vi "ExampleClient.vi"() -> ()   [LabVIEW 2017]
uses:
  jsonRPCwebservice/client/config.ctl
  <vilib>/rvi/Analysis/control/PID/Typedef/niFpgaPID_PIGains.ctl
  <vilib>/rvi/Analysis/control/PID/Typedef/niFpgaPID_OutputRange.ctl
  <vilib>/NI/PowerElectronicsControl/ActiveFrontEnd/AFE/PI_Settings.ctl
  <vilib>/NI/PowerElectronicsControl/Buck-Boost/RealTime/TuningParameters.ctl
  <vilib>/NI/PowerElectronicsControl/Buck-Boost/FPGA/contState.ctl
  Support/StreamClientState.ctl
  Controller/Support/StreamHeader.ctl
  Support/msg.ctl
  <userlib>/_SEH/Controls/CEH/CEH Actions.ctl
  <vilib>/NI/JSON Support for LabVIEW/JSON Data Classes/JSON String/JSON String.lvclass
  C:/Program Files (x86)/National Instruments/LabVIEW 2017/vi.lib/NI/JSON Support for LabVIEW/JSON Data Classes/JSON Datatype/JSON Null.lvclass
  <vilib>/NI/JSON Support for LabVIEW/JSON Data Classes/JSON Object/JSON Object.lvclass
  <vilib>/NI/JSON Support for LabVIEW/JSON Data Classes/JSON Numeric/JSON Numeric.lvclass
  Support/client_globals.vi
  jsonRPCwebservice/client/Request_int_JSON.vi
  <vilib>/NI/JSON Support for LabVIEW/JSON Data Classes/JSON Helper/To More Specific Type (Object).vi
  <vilib>/NI/JSON Support for LabVIEW/JSON Data Classes/JSON String/New JSON String.vi
  <vilib>/NI/JSON Support for LabVIEW/JSON Data Classes/JSON Helper/Parsing/Parse Value.vi
  <vilib>/NI/JSON Support for LabVIEW/JSON Data Classes/JSON Object/Get Value (Array).vi
  <vilib>/NI/JSON Support for LabVIEW/JSON Data Classes/JSON Array/Index Array XNode/index helper.vi
  <vilib>/NI/JSON Support for LabVIEW/JSON Data Classes/JSON Array/Index Array.vi
  <vilib>/NI/JSON Support for LabVIEW/JSON Data Classes/JSON Array/Index Array (JSON).vi
  <vilib>/NI/JSON Support for LabVIEW/JSON Data Classes/JSON Helper/To More Specific Type (Array).vi
  <vilib>/NI/JSON Support for LabVIEW/JSON Data Classes/JSON Array/Get Array Values as Strings.vi
  <vilib>/WebDAVClient/Simple Get File.vi
  <vilib>/NI/JSON Support for LabVIEW/JSON Data Classes/JSON Object/New JSON Object (Multi).vi
  <vilib>/NI/JSON Support for LabVIEW/JSON Data Classes/JSON Numeric/New JSON Numeric.vi
  <vilib>/NI/JSON Support for LabVIEW/JSON Data Classes/JSON Object/Get Value by Array (Object).vi
  <vilib>/NI/JSON Support for LabVIEW/JSON Data Classes/JSON Object/Get Value (Object).vi
  <vilib>/NI/JSON Support for LabVIEW/JSON Data Classes/JSON Datatype/JSON Null.lvclass
  <vilib>/NI/JSON Support for LabVIEW/JSON Data Classes/JSON Array/Index Array XNode/Index JSON Array.xnode
  <vilib>/NI/JSON Support for LabVIEW/JSON Data Classes/JSON Array/JSON Array.lvclass
  jsonRPCwebservice/client/JSON_RPC_client.lvlib
  <vilib>/WebDAVClient/NI_WebDAV.lvlib
  <vilib>/NI/JSON Support for LabVIEW/JSON Data Classes/JSON Helper/JSON Helper.lvclass
  <vilib>/NI/PowerElectronicsControl/ActiveFrontEnd/AFE/ActiveFrontEnd.lvlib
  <vilib>/NI/PowerElectronicsControl/Buck-Boost/FPGA/BuckBoost.lvlib
  <vilib>/NI/PowerElectronicsControl/Buck-Boost/RealTime/BuckBoostInterface.lvlib
panel:
  out "Load Current":dbl format="%_6g"
  out "BuckBoostEnabled":bool
  out "AFE_Enabled":bool
  out "Connected":bool
  out "Fault Registers":u64 format="%016x"
  out "VLoad":dbl format="%_6g"
  out "VDCLink":dbl format="%_6g"
  out "Detected Frequency":dbl format="%1_6g"
  out "locked":bool
  out "UnrecoverableSafeState":bool
  out "SafeState":bool
  out "Powered":bool
  out "EnableBuckBoost":bool
  out "EnableAFE":bool
  out "Precharge":bool
  out "Ready":bool
  out "Synchronize":bool
  out "TuneBuckBoost":bool
  out "TuneAFE":bool
  out "TunePLL":bool
  out "Idle":bool
  out "Initialize":bool
  in  "Connection":T1={"ip"="0.0.0.0", "port"=8001, "username"="admin", "password"=""}
  in  "Trace":string
  in  "Tab Control":T2(tab)
  in  "ClearSafeState":bool
  in  "ToEcho":string
  in  "CheckConnection":bool
  in  "GoToSafeState":bool
  in  "GetResourceUsage":bool
  in  "echo":bool
  out "logging":bool
  out "Waveforms":sgl[][](graph)
  in  "Stream":bool
  in  "StreamAndLog":bool
  in  "StopStreaming":bool
  in  "ForceTigger":bool
  in  "RefreshLogFiles":bool
  in  "Logs":i32(listbox)
  in  "Download":bool
  in  "BuckBoostSetpoint":dbl caption="Setpoint" format="%_6g"
  in  "TurnOffSystem":bool
  in  "SetBuckBoostSetpoint":bool
  in  "TurnOnSystem":bool
  in  "PrechargeSystem":bool
  in  "PLL Range":T3={"output high (Inf)"=inf, "output low (-Inf)"=-inf}
  in  "PLL Gains":T4 {"proportional gain" step=0.125}
  in  "SetPLL_Tune":bool
  in  "GoToTunePLL":bool
  in  "disableAFE":bool
  in  "enableAFE":bool
  in  "SetAFE_tune":bool
  in  "GoToTuneAFE":bool
  in  "IQ_to_VQ":T5={"gains"={"proportional gain"=0.0, "integral gain"=0.0}, "output range"={"output high (Inf)"=inf, "output low (-Inf)"=-inf}, "PI_state"=enum."idle", "reset"=FALSE, "manual"=0.0} {"gains"."proportional gain" step=0.125}
  in  "ID_to_VD":T5={"gains"={"proportional gain"=0.0, "integral gain"=0.0}, "output range"={"output high (Inf)"=inf, "output low (-Inf)"=-inf}, "PI_state"=enum."idle", "reset"=FALSE, "manual"=0.0} {"gains"."proportional gain" step=0.125}
  in  "VDCLinkToPower":T5={"gains"={"proportional gain"=0.0, "integral gain"=0.0}, "output range"={"output high (Inf)"=inf, "output low (-Inf)"=-inf}, "PI_state"=enum."idle", "reset"=FALSE, "manual"=0.0} {"gains"."proportional gain" step=0.125}
  in  "disableBuckBoost":bool
  in  "SetBuckBoostTune":bool
  in  "GoToTuneBuckBoost":bool
  in  "CompleteTuning":bool
  in  "BuckBoostTune":T6 caption="Buck-Boost Tune" {"gains"."proportional gain" step=0.125}
  in  "enableBuckBoost":bool
  in  "Exit":bool
  # "Tuning"
  # "rad/sec"
  # "V"
  # "V"
  # "Amps"
  # "Amps"
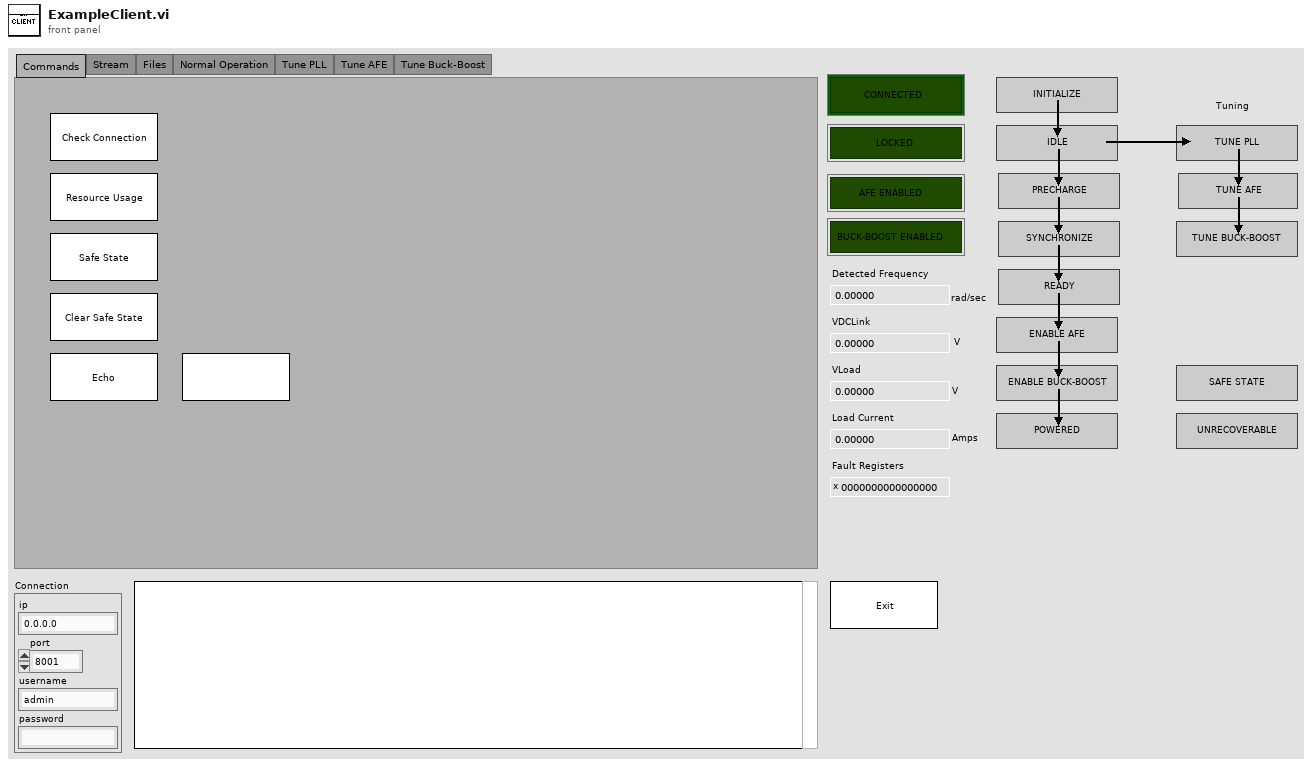
[diagram p1: front panel]
types:
  T1 = typedef "JSON_RPC_client.lvlib/config.ctl" = cluster{"ip":string, "port":i32, "username":string, "password":string}
  T2 = enum32{"Commands", "Stream", "Files", "Normal Operation", "Tune PLL", "Tune AFE", "Tune Buck-Boost"}
  T3 = typedef "niFpgaPID_OutputRange.ctl" = cluster{"output high (Inf)":sgl, "output low (-Inf)":sgl}
  T4 = typedef "niFpgaPID_PIGains.ctl" = cluster{"proportional gain":sgl, "integral gain":sgl}
  T5 = typedef "ActiveFrontEnd.lvlib/PI_Settings.ctl" = cluster{"gains":T4, "output range":T3, "PI_state":enum8{"idle", "normal", "manual", "perturbance"}, "reset":bool, "manual":sgl}
  T6 = typedef "BuckBoostInterface.lvlib/TuningParameters.ctl" = cluster{"gains":T4, "manualInput":sgl, "rampRate":sgl, "pertAmp":sgl, "pertFreq":sgl, "controlFreq":sgl, "state":T7}
  T7 = typedef "BuckBoost.lvlib/contState.ctl" = enum16{"disabled", "manual", "normal", "perturb"}
  T8 = typedef "msg.ctl" = cluster{"cmd":string, "parameters":variant}
  T9 = typedef "StreamHeader.ctl" = cluster{"Channels":string[], "SampleRate":i32}
  T10 = typedef "StreamClientState.ctl" = enum16{"Initialize", "Idle", "ConnectAndOpen", "Connecting", "ReadHeader", "Streaming", "Disconnecting"}
  T11 = enum8{"Enabled", "Disabled", "Disabled and Grayed Out"}
  T12 = typedef "JSON_RPC_client.lvlib/reference.ctl" = cluster{"client handle":T13, "url":string}
  T13 = typedef "LabVIEWHTTPClient.lvlib/ClientHandle.ctl" = refnum<k1>
  T14 = typedef "StateMsg.ctl" = cluster{"State":string, "locked":bool, "DetectedFrequency":dbl, "VDCLink":dbl, "VLoad":dbl, "FaultRegisters":u64, "afeEnabled":bool, "buckboostEnabled":bool, "LoadCurrent":dbl}
  T15 = typedef "SEH Notification Info.ctl" = cluster{"Priority":i32, "Occurrences":i32, "First Occurrence":timestamp}
  T16 = typedef "CEH Actions.ctl" = enum16{"Log", "Display Error Message", "Safe State", "Shutdown"}
  T17 = enum16{"open", "open or create", "create or replace", "create", "open (read-only)"}
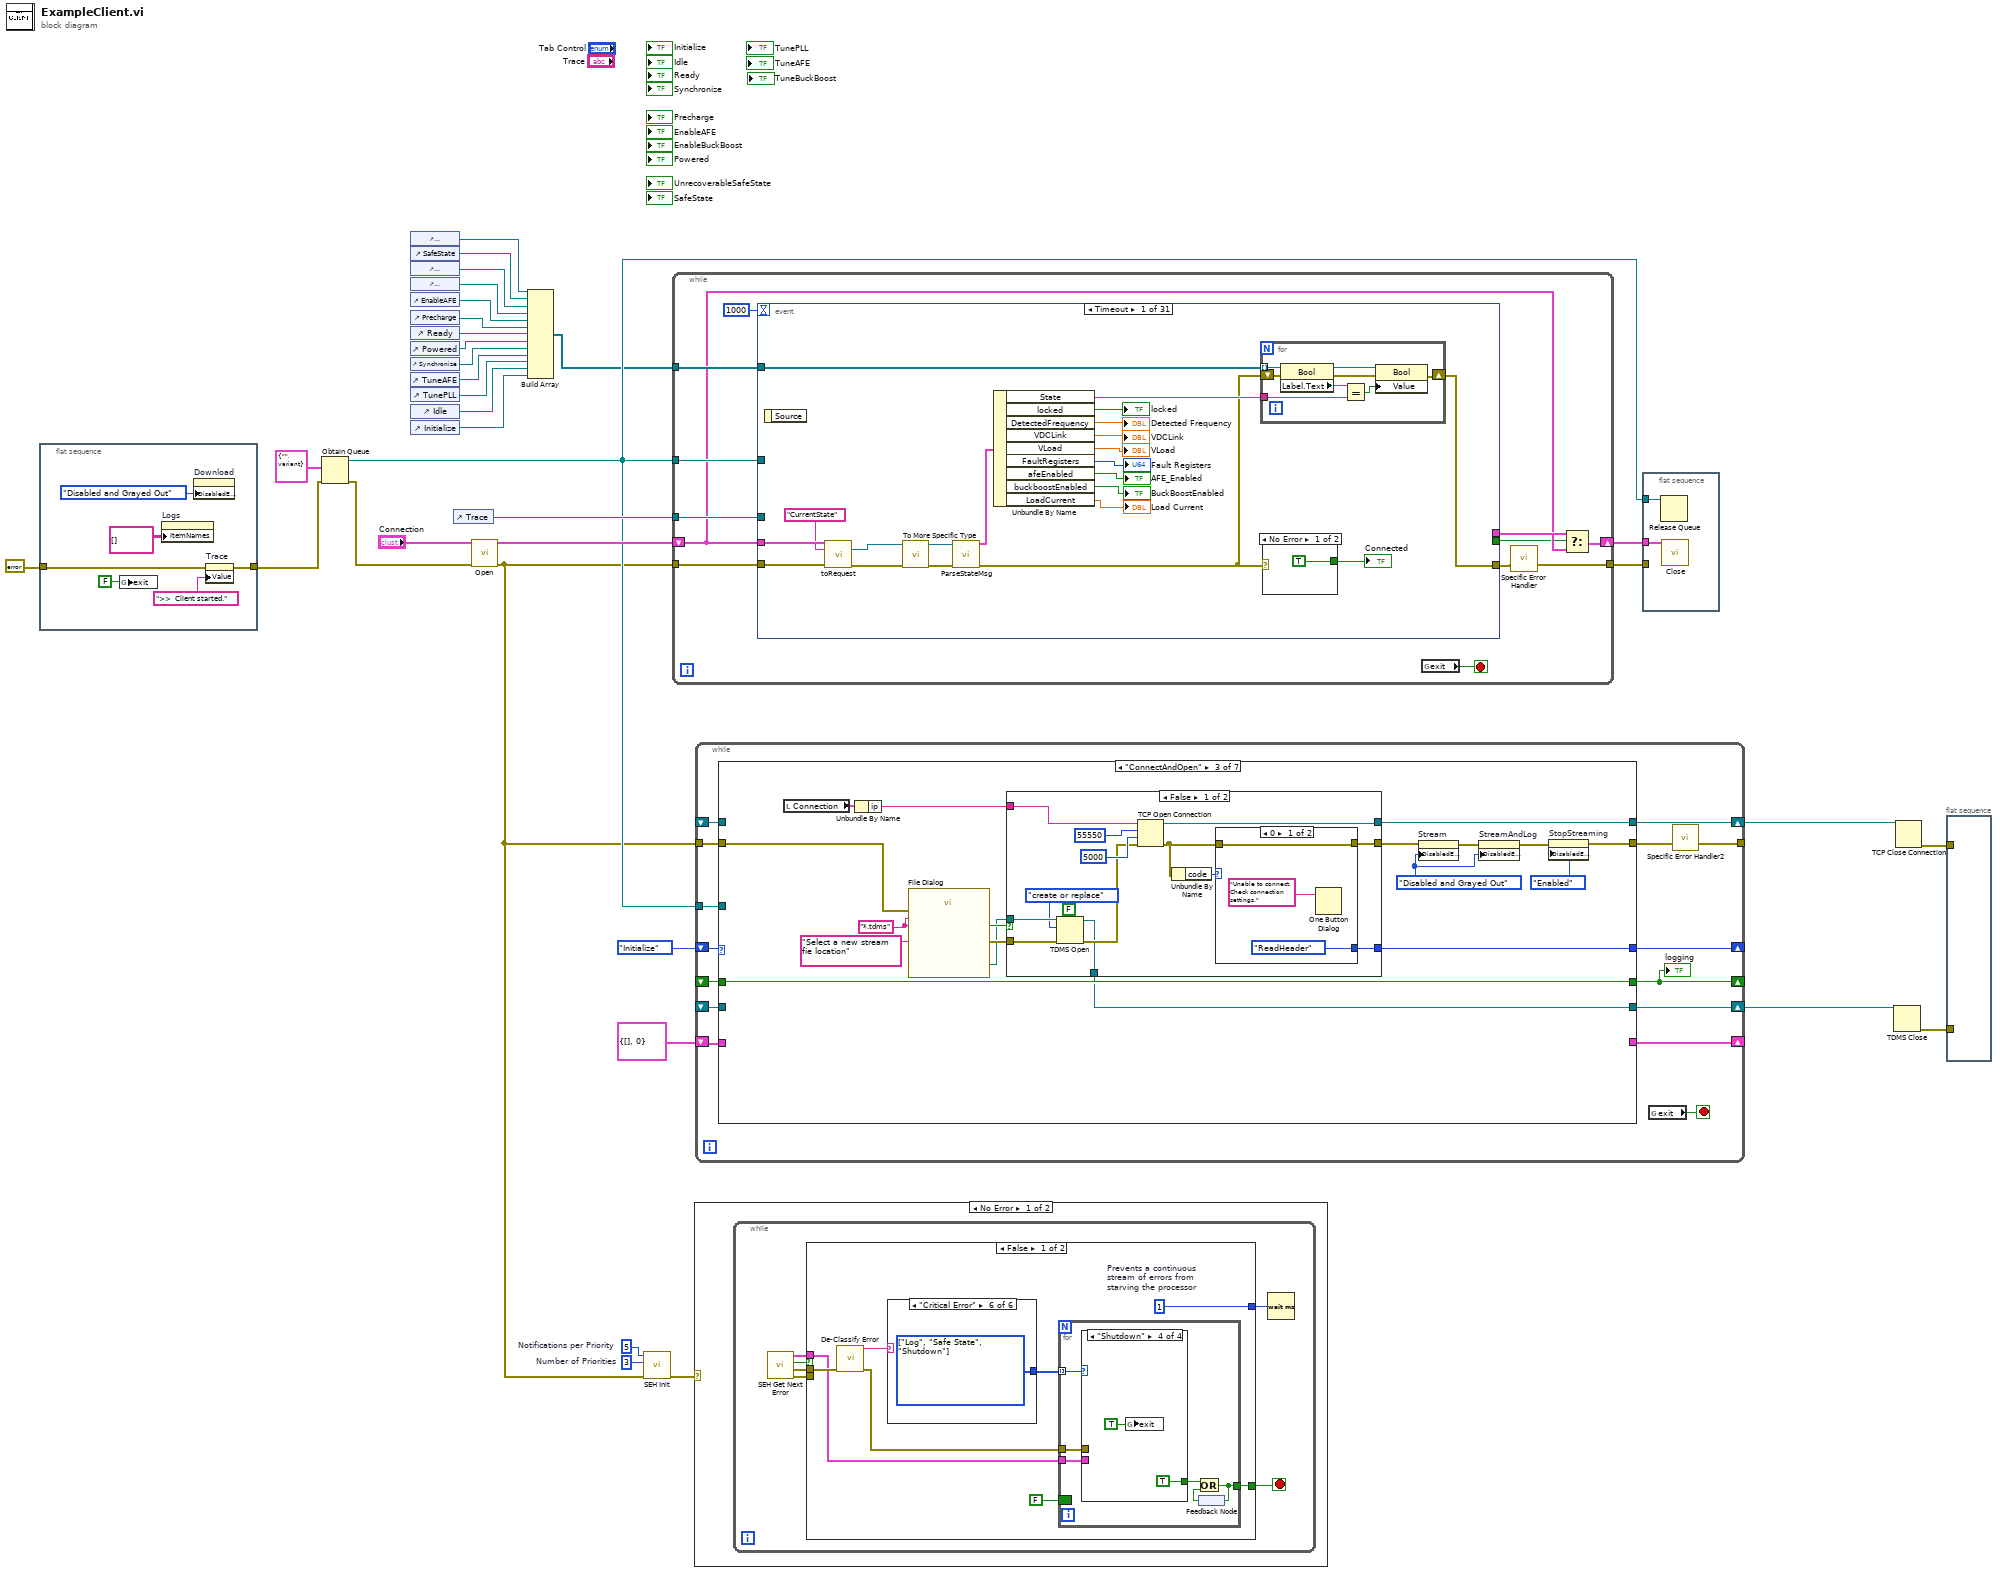
[diagram p0: block diagram]
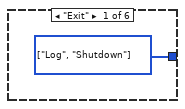
[diagram p2: hidden frame]
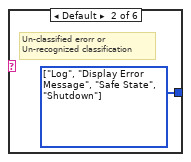
[diagram p3: hidden frame]
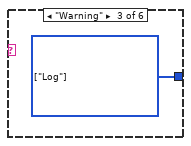
[diagram p4: hidden frame]
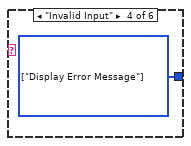
[diagram p5: hidden frame]
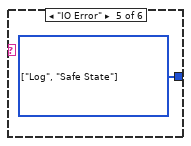
[diagram p6: hidden frame]
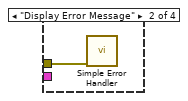
[diagram p8: hidden frame]
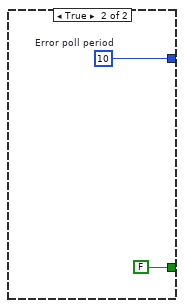
[diagram p10: hidden frame]
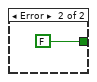
[diagram p12: hidden frame]
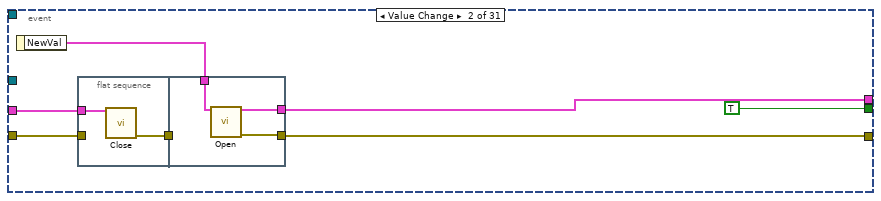
[diagram p13: hidden frame]
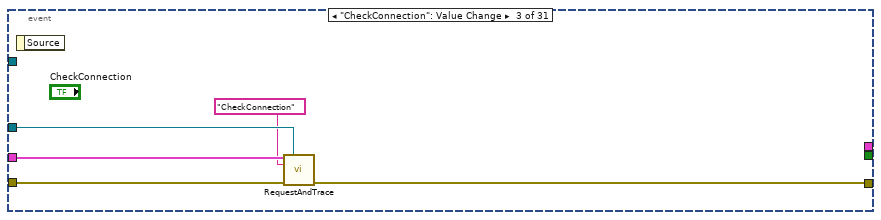
[diagram p14: hidden frame]
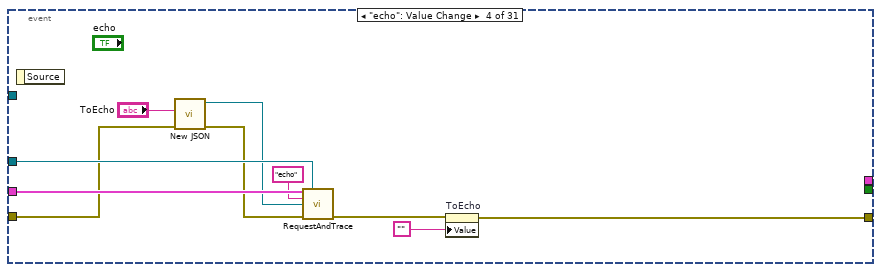
[diagram p15: hidden frame]
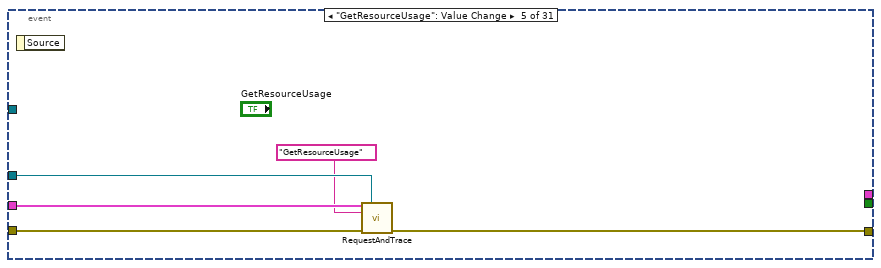
[diagram p16: hidden frame]
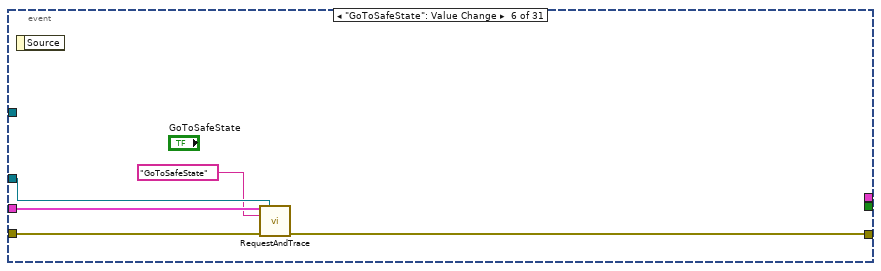
[diagram p17: hidden frame]
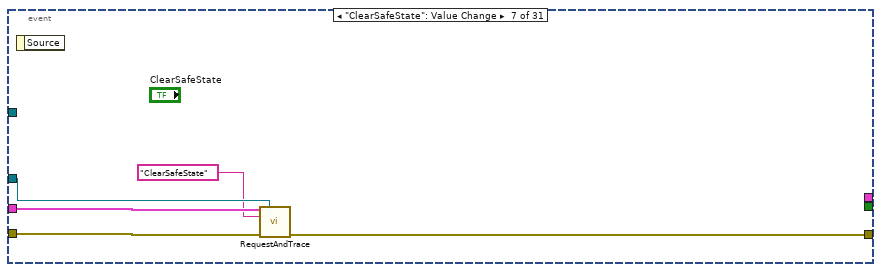
[diagram p18: hidden frame]
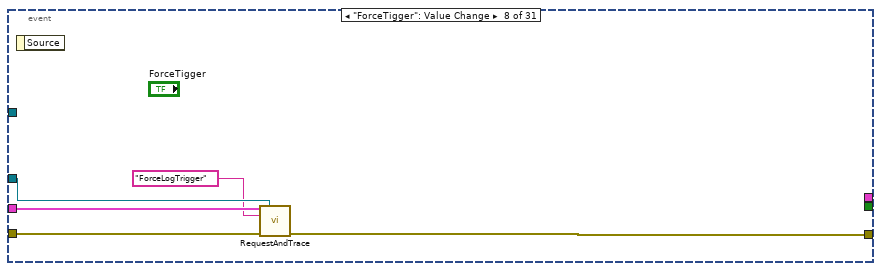
[diagram p19: hidden frame]
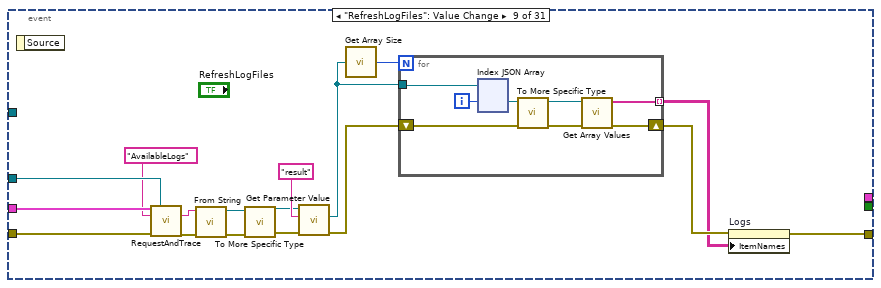
[diagram p20: hidden frame]
diagram:
  w23 = 3  # Number of Priorities
  w22 = 5  # Notifications per Priority
  n1 = flat-sequence {
    tunnel: errorcluster {"status"=FALSE, "code"=0, "source"=""} ("error in (no error)") -> [w38]
    tunnel: [w37] -> w27
    frame #0 {
      n2 = global write "client_globals.vi" "exit"(FALSE ("exit")) -> ()
      n3 = property on="Logs" class="MCListbox (strict)"("ItemNames"=string[][] [] ("Item Names")) -> ()  [unwired: 2 in, 2 out]
      n4 = property on="Download" class="Bool"("DisabledEnum"=T11."Disabled and Grayed Out" ("Disabled")) -> ()  [unwired: 2 in, 2 out]
      n5 = property on="Trace" class="Str"(error in=w38, "Value"=">>  Client started." ("Trace")) -> (error out=w37:errorcluster)  [unwired: 1 in, 1 out]
    }
  }
  n6 = Obtain Queue(element data type=T8 {"cmd"="", "parameters"=variant} ("msg"), error in (no error)=w27) -> (queue out=w25:refnum<queue>, error out=w26:errorcluster)  [unwired: 3 in, 1 out]
  n7 = control-ref of="UnrecoverableSafeState"() -> (w15:refnum<vi>)
  n8 = control-ref of="SafeState"() -> (w14:refnum<vi>)
  n9 = control-ref of="TuneBuckBoost"() -> (w13:refnum<vi>)
  n10 = control-ref of="EnableBuckBoost"() -> (w12:refnum<vi>)
  n11 = control-ref of="EnableAFE"() -> (w11:refnum<vi>)
  n12 = control-ref of="Precharge"() -> (w10:refnum<vi>)
  n13 = control-ref of="Ready"() -> (w9:refnum<vi>)
  n14 = control-ref of="Powered"() -> (w8:refnum<vi>)
  n15 = control-ref of="Synchronize"() -> (w7:refnum<vi>)
  n16 = control-ref of="TuneAFE"() -> (w6:refnum<vi>)
  n17 = control-ref of="TunePLL"() -> (w5:refnum<vi>)
  n18 = control-ref of="Idle"() -> (w4:refnum<vi>)
  n19 = control-ref of="Initialize"() -> (w3:refnum<vi>)
  n20 = control-ref of="Trace"() -> (w29:refnum<vi>)
  n21 = call "Open.vi"("config"="Connection", "error in (no error)"=w26) -> ("reference"=w32:T12, "error out"=w20:errorcluster)  [unwired: 12 in]
  n22 = Build Array(w15, w14, w13, w12, w11, w10, w9, w8, w7, w6, w5, w4, w3) -> (w2:refnum<vi>[])
  n23 = call <userlib>:"SEH Init.vi"("error in (no error)"=w20, "Number of Priorities"=w23, "Notifications per Priority"=w22) -> ("error out"=w21:errorcluster)  [unwired: 8 in]
  n24 = while {
    tunnel: w29 -> [w47]
    tunnel: w25 -> [w46]
    tunnel: w20 -> [w52]
    tunnel: [w48] -> w30
    tunnel: w2 -> [w45]
    shift-right: [w44] -> w1
    shift-left: w32 -> [w42]
    stop <- w50 stop-if-true
    n25 = event shown="[0] Timeout" {
      selector: _ -> [_ _ _ _ _ _ _ _ _ _ _ _ _ _ _ _ _ _ _ _ _ _ _ _ _ _ _ _ _ _ _]
      dyn-events: _ -> [_ _ _ _ _ _ _ _ _ _ _ _ _ _ _ _ _ _ _ _ _ _ _ _ _ _ _ _ _ _ _]
      timeout: 1000 -> [_ _ _ _ _ _ _ _ _ _ _ _ _ _ _ _ _ _ _ _ _ _ _ _ _ _ _ _ _ _ _]
      tunnel: w42 -> [w72 w90 w98 w110 w115 w120 w125 w130 w147 _ _ _ _ _ w216 w221 w226 w231 w236 w241 w257 w265 w269 w288 w293 w298 w303 w308 w316 w322 _]
      tunnel: w52 -> [w73 w89 w100 w103 w114 w119 w124 w129 w146 w163 w183 w198 w204 w211 w217 w222 w227 w232 w237 w242 w246 w261 w270 w284 w290 w295 w300 w305 w313 w319 _]
      tunnel: [w67 w85 w99 w107 w112 w117 w122 w127 w144 w164 w176 w197 w201 w207 w215 w220 w225 w230 w235 w240 w256 w264 w268 w287 w292 w297 w302 w307 w315 w321 errorcluster {"status"=TRUE, "code"=-1, "source"="User selected exit."} ("error out")] -> w49
      tunnel: w47 -> [_ _ w97 w109 w113 w118 w123 w128 w145 _ _ _ w200 w209 w214 w219 w224 w229 w234 w239 w255 w263 w267 w286 w291 w296 w301 w306 w314 w320 _]
      tunnel: w46 -> [_ _ _ _ _ _ _ _ _ _ _ w199 w205 w212 _ _ _ _ _ _ _ _ _ _ _ _ _ _ _ _ _]
      tunnel: w45 -> [w68 _ _ _ _ _ _ _ _ _ _ _ _ _ _ _ _ _ _ _ _ _ _ _ _ _ _ _ _ _ _]
      tunnel: [_ w86 _ _ _ _ _ _ _ _ _ _ _ _ _ _ _ _ _ _ _ _ _ _ _ _ _ _ _ _ _] -> w43
      tunnel: [_ TRUE _ _ _ _ _ _ _ _ _ _ _ _ _ _ _ _ _ _ _ _ _ _ _ _ _ _ _ _ _] -> w41
      event Timeout {
        n26 = event-data() -> ()  [unwired: 1 in, 1 out]
        n27 = call-poly "toRequest.vi"("reference in"=w72, "method"="CurrentState" ("resulting string"), "error in (no error)"=w73) -> ("response"=w70:refnum<class "JSON Null.lvclass">, "error out"=w69:errorcluster)  [unwired: 10 in, 1 out]
        n28 = call-poly <vilib>:"To More Specific Type.vi"("error in (no error)"=w69, "JSON Datatype in"=w70) -> ("error out"=w65:errorcluster, "JSON Datatype out"=w64:refnum<class "JSON Object.lvclass">)  [unwired: 8 in]
        n29 = call "ParseStateMsg.vi"("StateMsg"=w64, "error in"=w65) -> ("StateMsg"=w63:T14, "error out"=w61:errorcluster)  [unwired: 12 in]
        n30 = Unbundle By Name(w63) -> ("State"=w62:string, "locked"=→"locked":bool, "DetectedFrequency"=→"Detected Frequency":dbl, "VDCLink"=→"VDCLink":dbl, "VLoad"=→"VLoad":dbl, "FaultRegisters"=→"Fault Registers":u64, "afeEnabled"=→"AFE_Enabled":bool, "buckboostEnabled"=→"BuckBoostEnabled":bool, "LoadCurrent"=→"Load Current":dbl)
        n31 = for {
          tunnel: w62 -> [w81]
          tunnel: w68 -> [w83] mode=indexing
          shift-right: [w77] -> w67
          shift-left: w61 -> [w78]
          n32 = property class="Bool"(reference=w83, error in=w78) -> (reference out=w80:refnum<vi>, error out=w76:errorcluster, "Label.Text"=w82:string)
          n33 = Equal?(x=w82, y=w81) -> (x = y?=w79:bool)
          n34 = property class="Bool"(reference=w80, error in=w76, "Value"=w79) -> (error out=w77:errorcluster)  [unwired: 1 out]
        }
        n35 = case shown="No Error" w61 {
          tunnel: [TRUE FALSE] -> w66
          frame No Error {
          }
          frame Error {
          }
        }
        "Connected" <- w66
      }
      event Value Change {
        n36 = event-data() -> ("NewVal"=w87:T1)  [unwired: 1 in]
        n37 = flat-sequence {
          tunnel: w90 -> [w92]
          tunnel: w89 -> [_]
          tunnel: [w91] -> w88
          tunnel: w88 -> [_]
          tunnel: w87 -> [w95]
          tunnel: [w94] -> w85
          tunnel: [w93] -> w86
          frame #0 {
            n38 = call "Close.vi"("reference in"=w92) -> ("error out"=w91:errorcluster)  [unwired: 14 in]
          }
          frame #1 {
            n39 = call "Open.vi"("config"=w95) -> ("reference"=w93:T12, "error out"=w94:errorcluster)  [unwired: 13 in]
          }
        }
      }
      event "CheckConnection": Value Change {
        n40 = event-data() -> ()  [unwired: 1 in, 1 out]
        n41 = call "RequestAndTrace.vi"("JSONRef in"=w98, "TraceRef"=w97, "method"="CheckConnection" ("resulting string"), "error in (no error)"=w100) -> ("error out"=w99:errorcluster)  [unwired: 9 in, 2 out]
      }
      event "echo": Value Change {
        n42 = event-data() -> ()  [unwired: 1 in, 1 out]
        n43 = call-poly <vilib>:"New JSON.vi"("error in (no error)"=w103, "value"="ToEcho") -> ("error out"=w102:errorcluster, "JSON String out"=w101:refnum<class "JSON String.lvclass">)  [unwired: 8 in]
        n44 = call "RequestAndTrace.vi"("JSONRef in"=w110, "TraceRef"=w109, "method"="echo" ("resulting string"), "params"=w101, "error in (no error)"=w102) -> ("error out"=w108:errorcluster)  [unwired: 8 in, 2 out]
        n45 = property on="ToEcho" class="Str"(error in=w108, "Value"="") -> (error out=w107:errorcluster)  [unwired: 1 in, 1 out]
      }
      event "GetResourceUsage": Value Change {
        n46 = event-data() -> ()  [unwired: 1 in, 1 out]
        n47 = call "RequestAndTrace.vi"("JSONRef in"=w115, "TraceRef"=w113, "method"="GetResourceUsage" ("resulting string"), "error in (no error)"=w114) -> ("error out"=w112:errorcluster)  [unwired: 9 in, 2 out]
      }
      event "GoToSafeState": Value Change {
        n48 = event-data() -> ()  [unwired: 1 in, 1 out]
        n49 = call "RequestAndTrace.vi"("JSONRef in"=w120, "TraceRef"=w118, "method"="GoToSafeState" ("resulting string"), "error in (no error)"=w119) -> ("error out"=w117:errorcluster)  [unwired: 9 in, 2 out]
      }
      event "ClearSafeState": Value Change {
        n50 = event-data() -> ()  [unwired: 1 in, 1 out]
        n51 = call "RequestAndTrace.vi"("JSONRef in"=w125, "TraceRef"=w123, "method"="ClearSafeState" ("resulting string"), "error in (no error)"=w124) -> ("error out"=w122:errorcluster)  [unwired: 9 in, 2 out]
      }
      event "ForceTigger": Value Change {
        n52 = event-data() -> ()  [unwired: 1 in, 1 out]
        n53 = call "RequestAndTrace.vi"("JSONRef in"=w130, "TraceRef"=w128, "method"="ForceLogTrigger" ("resulting string"), "error in (no error)"=w129) -> ("error out"=w127:errorcluster)  [unwired: 9 in, 2 out]
      }
      event "RefreshLogFiles": Value Change {
        n54 = event-data() -> ()  [unwired: 1 in, 1 out]
        n55 = call "RequestAndTrace.vi"("JSONRef in"=w147, "TraceRef"=w145, "method"="AvailableLogs" ("resulting string"), "error in (no error)"=w146) -> ("reponse"=w141:string, "error out"=w142:errorcluster)  [unwired: 9 in, 1 out]
        n56 = call <vilib>:"From String.vi"("error in (no error)"=w142, "JSON String"=w141) -> ("error out"=w134:errorcluster, "JSON out"=w133:refnum<class "JSON Null.lvclass">)  [unwired: 8 in]
        n57 = call-poly <vilib>:"To More Specific Type.vi"("error in (no error)"=w134, "JSON Datatype in"=w133) -> ("error out"=w131:errorcluster, "JSON Datatype out"=w132:refnum<class "JSON Object.lvclass">)  [unwired: 8 in]
        n58 = call-poly <vilib>:"Get Parameter Value.vi"("error in (no error)"=w131, "key"="result" ("Parameter Name"), "JSON Object in"=w132) -> ("error out"=w139:errorcluster, "value"=w136:refnum<class "JSON Array.lvclass">)  [unwired: 7 in]
        n59 = call <vilib>:"Get Array Size.vi"("JSON Array in"=w136) -> ("size(s)"=w137:i32)
        n60 = for {
          N: w137 -> [_]
          tunnel: w136 -> [w155]
          shift-right: [w149] -> w138
          shift-left: w139 -> [w152]
          tunnel: [w148] -> w135 mode=indexing
          i -> [w154]
          n61 = xnode "Index JSON Array"("index"=w154, "JSON Array In"=w155) -> ("element"=w153:refnum<class "JSON Null.lvclass">)  [unwired: 1 in, 1 out]
          n62 = call-poly <vilib>:"To More Specific Type.vi"("error in (no error)"=w152, "JSON Datatype in"=w153) -> ("error out"=w150:errorcluster, "JSON Datatype out"=w151:refnum<class "JSON Array.lvclass">)  [unwired: 8 in]
          n63 = call-poly <vilib>:"Get Array Values.vi"("error in (no error)"=w150, "JSON Array in"=w151) -> ("error out"=w149:errorcluster, "values"=w148:string[])  [unwired: 8 in]
        }
        n64 = property on="Logs" class="MCListbox (strict)"(error in=w138, "ItemNames"=w135) -> (error out=w144:errorcluster)  [unwired: 1 in, 1 out]
      }
      event "Logs": Value Change {
        n65 = event-data() -> ()  [unwired: 1 in, 1 out]
        n66 = case shown="-1" "Logs" {
          tunnel: w163 -> [w167 w168]
          tunnel: [w167 w168] -> w162
          tunnel: [T11."Enabled" ("Disabled") T11."Disabled and Grayed Out" ("Disabled")] -> w161
          frame Default {
          }
          frame -1 {
          }
        }
        n67 = property on="Download" class="Bool"(error in=w162, "DisabledEnum"=w161) -> (error out=w164:errorcluster)  [unwired: 1 in, 1 out]
      }
      event "Download": Value Change {
        # "http[s]://hostname[:port][/files][/directory/subdirectory]/filename"
        n68 = event-data() -> ()  [unwired: 1 in, 1 out]
        n69 = property on="Logs" class="MCListbox (strict)"() -> ("ItemNames"=w181:string[][])  [unwired: 2 in, 2 out]
        n70 = local read "Connection"() -> (w170:T1)
        n71 = property on="Logs" class="MCListbox (strict)"(error in=w183) -> (error out=w175:errorcluster, "FocusRow"=w182:i32)  [unwired: 1 in, 1 out]
        n72 = Index Array(array=w181, index (row)=w182, index (col)=0 ("index")) -> (element=w173:string)
        n73 = Unbundle By Name(w170) -> ("ip"=w179:string, "username"=w178:string, "password"=w177:string)
        n74 = call "File Dialog2"("error in"=w175) -> ("selected path"=w174:path, "cancelled"=w171:bool, "error out"=w172:errorcluster)  [unwired: 11 in, 1 out]
        n75 = case shown="False" w171 {
          tunnel: w179 -> [w193 _]
          tunnel: w178 -> [w190 _]
          tunnel: w177 -> [w189 _]
          tunnel: [w188 w195] -> w176
          tunnel: w174 -> [w187 _]
          tunnel: w173 -> [w186 _]
          tunnel: w172 -> [w184 w195]
          frame False {
            n76 = Build Path(base path=w187, name or relative path=w186) -> (appended path=w185:path)
            n77 = Concatenate Strings("http://" ("string"), w193, "/files/home/lvuser/logs/" ("string"), w186) -> (w191:string)
            n78 = call-poly <vilib>:"Simple Get.vi"("remote file uri"=w191, "username"=w190, "password"=w189, "local file path"=w185, "error in (no error)"=w184) -> ("error out"=w188:errorcluster)  [unwired: 9 in, 1 out]
          }
          frame True {
          }
        }
      }
      event "Stream": Value Change {
        n79 = event-data() -> ()  [unwired: 1 in, 1 out]
        n80 = Enqueue Element(queue=w199, element=T8 {"cmd"="StartStream", "parameters"=variant}, error in (no error)=w198) -> (error out=w197:errorcluster)  [unwired: 1 in, 2 out]
      }
      event "StreamAndLog": Value Change {
        n81 = event-data() -> ()  [unwired: 1 in, 1 out]
        n82 = Enqueue Element(queue=w205, element=T8 {"cmd"="StartStreamAndLog", "parameters"=variant}, error in (no error)=w204) -> (error out=w202:errorcluster)  [unwired: 1 in, 2 out]
        n83 = call "ToTrace.vi"("ToTrace"="Stream and log started.", "TraceRef"=w200, "error in (no error)"=w202) -> ("error out"=w201:errorcluster)  [unwired: 12 in]
      }
      event "StopStreaming": Value Change {
        n84 = event-data() -> ()  [unwired: 1 in, 1 out]
        n85 = Enqueue Element(queue=w212, element=T8 {"cmd"="StopStream", "parameters"=variant}, error in (no error)=w211) -> (error out=w210:errorcluster)  [unwired: 1 in, 2 out]
        n86 = call "ToTrace.vi"("ToTrace"="Streaming stopped.", "TraceRef"=w209, "error in (no error)"=w210) -> ("error out"=w207:errorcluster)  [unwired: 12 in]
      }
      event "GoToTuneAFE": Value Change {
        n87 = event-data() -> ()  [unwired: 1 in, 1 out]
        n88 = call "RequestAndTrace.vi"("JSONRef in"=w216, "TraceRef"=w214, "method"="GoToTuneAFE" ("resulting string"), "error in (no error)"=w217) -> ("error out"=w215:errorcluster)  [unwired: 9 in, 2 out]
      }
      event "GoToTunePLL": Value Change {
        n89 = event-data() -> ()  [unwired: 1 in, 1 out]
        n90 = call "RequestAndTrace.vi"("JSONRef in"=w221, "TraceRef"=w219, "method"="GoToTunePLL" ("resulting string"), "error in (no error)"=w222) -> ("error out"=w220:errorcluster)  [unwired: 9 in, 2 out]
      }
      event "GoToTuneBuckBoost": Value Change {
        n91 = event-data() -> ()  [unwired: 1 in, 1 out]
        n92 = call "RequestAndTrace.vi"("JSONRef in"=w226, "TraceRef"=w224, "method"="GoToTuneBuckBoost" ("resulting string"), "error in (no error)"=w227) -> ("error out"=w225:errorcluster)  [unwired: 9 in, 2 out]
      }
      event "TurnOnSystem": Value Change {
        n93 = event-data() -> ()  [unwired: 1 in, 1 out]
        n94 = call "RequestAndTrace.vi"("JSONRef in"=w231, "TraceRef"=w229, "method"="TurnOnSystem" ("resulting string"), "error in (no error)"=w232) -> ("error out"=w230:errorcluster)  [unwired: 9 in, 2 out]
      }
      event "TurnOffSystem": Value Change {
        n95 = event-data() -> ()  [unwired: 1 in, 1 out]
        n96 = call "RequestAndTrace.vi"("JSONRef in"=w236, "TraceRef"=w234, "method"="TurnOffSystem" ("resulting string"), "error in (no error)"=w237) -> ("error out"=w235:errorcluster)  [unwired: 9 in, 2 out]
      }
      event "PrechargeSystem": Value Change {
        n97 = event-data() -> ()  [unwired: 1 in, 1 out]
        n98 = call "RequestAndTrace.vi"("JSONRef in"=w241, "TraceRef"=w239, "method"="PrechargeSystem" ("resulting string"), "error in (no error)"=w242) -> ("error out"=w240:errorcluster)  [unwired: 9 in, 2 out]
      }
      event "SetPLL_Tune": Value Change {
        n99 = event-data() -> ()  [unwired: 1 in, 1 out]
        n100 = call <vilib>:"From Variant.vi"("error in (no error)"=w246, "Variant"="PLL Range") -> ("error out"=w254:errorcluster, "JSON out"=w253:refnum<class "JSON Null.lvclass">)  [unwired: 8 in]
        n101 = call <vilib>:"From Variant.vi"("error in (no error)"=w254, "Variant"="PLL Gains") -> ("error out"=w248:errorcluster, "JSON out"=w252:refnum<class "JSON Null.lvclass">)  [unwired: 8 in]
        n102 = Build Array(w253, w252) -> (w251:refnum<class "JSON Null.lvclass">[])
        n103 = call-poly <vilib>:"New JSON.vi"("keys"=string[] ["PLLrange", "PLLgains"], "error in (no error)"=w248, "values"=w251) -> ("error out"=w245:errorcluster, "JSON Object out"=w244:refnum<class "JSON Object.lvclass">)  [unwired: 7 in]
        n104 = call "RequestAndTrace.vi"("JSONRef in"=w257, "TraceRef"=w255, "method"="SetPLL_Tune" ("resulting string"), "params"=w244, "error in (no error)"=w245) -> ("error out"=w256:errorcluster)  [unwired: 8 in, 2 out]
      }
      event "SetBuckBoostSetpoint": Value Change {
        n105 = event-data() -> ()  [unwired: 1 in, 1 out]
        n106 = call-poly <vilib>:"New JSON.vi"("error in (no error)"=w261, "value"="BuckBoostSetpoint") -> ("error out"=w259:errorcluster, "JSON String out"=w260:refnum<class "JSON Numeric.lvclass">)  [unwired: 8 in]
        n107 = call "RequestAndTrace.vi"("JSONRef in"=w265, "TraceRef"=w263, "method"="SetBuckBoostSetpoint" ("resulting string"), "params"=w260, "error in (no error)"=w259) -> ("error out"=w264:errorcluster)  [unwired: 8 in, 2 out]
      }
      event "CompleteTuning": Value Change {
        n108 = event-data() -> ()  [unwired: 1 in, 1 out]
        n109 = call "RequestAndTrace.vi"("JSONRef in"=w269, "TraceRef"=w267, "method"="CompleteTuning" ("resulting string"), "error in (no error)"=w270) -> ("error out"=w268:errorcluster)  [unwired: 9 in, 2 out]
      }
      event "SetAFE_tune": Value Change {
        n110 = event-data() -> ()  [unwired: 1 in, 1 out]
        n111 = call <vilib>:"From Variant.vi"("error in (no error)"=w284, "Variant"="ID_to_VD") -> ("error out"=w283:errorcluster, "JSON out"=w279:refnum<class "JSON Null.lvclass">)  [unwired: 8 in]
        n112 = call <vilib>:"From Variant.vi"("error in (no error)"=w283, "Variant"="IQ_to_VQ") -> ("error out"=w281:errorcluster, "JSON out"=w278:refnum<class "JSON Null.lvclass">)  [unwired: 8 in]
        n113 = call <vilib>:"From Variant.vi"("error in (no error)"=w281, "Variant"="VDCLinkToPower") -> ("error out"=w274:errorcluster, "JSON out"=w277:refnum<class "JSON Null.lvclass">)  [unwired: 8 in]
        n114 = Build Array(w279, w278, w277) -> (w276:refnum<class "JSON Null.lvclass">[])
        n115 = call-poly <vilib>:"New JSON.vi"("keys"=string[] ["ID_to_VD", "IQ_to_VQ", "VDCLinkToPower"], "error in (no error)"=w274, "values"=w276) -> ("error out"=w273:errorcluster, "JSON Object out"=w272:refnum<class "JSON Object.lvclass">)  [unwired: 7 in]
        n116 = call "RequestAndTrace.vi"("JSONRef in"=w288, "TraceRef"=w286, "method"="SetAFE_tune" ("resulting string"), "params"=w272, "error in (no error)"=w273) -> ("error out"=w287:errorcluster)  [unwired: 8 in, 2 out]
      }
      event "enableAFE": Value Change {
        n117 = event-data() -> ()  [unwired: 1 in, 1 out]
        n118 = call "RequestAndTrace.vi"("JSONRef in"=w293, "TraceRef"=w291, "method"="enableAfe" ("resulting string"), "error in (no error)"=w290) -> ("error out"=w292:errorcluster)  [unwired: 9 in, 2 out]
      }
      event "disableAFE": Value Change {
        n119 = event-data() -> ()  [unwired: 1 in, 1 out]
        n120 = call "RequestAndTrace.vi"("JSONRef in"=w298, "TraceRef"=w296, "method"="disableAfe" ("resulting string"), "error in (no error)"=w295) -> ("error out"=w297:errorcluster)  [unwired: 9 in, 2 out]
      }
      event "enableBuckBoost": Value Change {
        n121 = event-data() -> ()  [unwired: 1 in, 1 out]
        n122 = call "RequestAndTrace.vi"("JSONRef in"=w303, "TraceRef"=w301, "method"="enableBuckBoost" ("resulting string"), "error in (no error)"=w300) -> ("error out"=w302:errorcluster)  [unwired: 9 in, 2 out]
      }
      event "disableBuckBoost": Value Change {
        n123 = event-data() -> ()  [unwired: 1 in, 1 out]
        n124 = call "RequestAndTrace.vi"("JSONRef in"=w308, "TraceRef"=w306, "method"="disableBuckBoost" ("resulting string"), "error in (no error)"=w305) -> ("error out"=w307:errorcluster)  [unwired: 9 in, 2 out]
      }
      event "SetBuckBoostTune": Value Change {
        n125 = event-data() -> ()  [unwired: 1 in, 1 out]
        n126 = call <vilib>:"From Variant.vi"("error in (no error)"=w313, "Variant"="BuckBoostTune") -> ("error out"=w311:errorcluster, "JSON out"=w310:refnum<class "JSON Null.lvclass">)  [unwired: 8 in]
        n127 = call "RequestAndTrace.vi"("JSONRef in"=w316, "TraceRef"=w314, "method"="SetBuckBoostTune" ("resulting string"), "params"=w310, "error in (no error)"=w311) -> ("error out"=w315:errorcluster)  [unwired: 8 in, 2 out]
      }
      event "Tab Control": Value Change {
        n128 = event-data() -> ("NewVal"=w318:T2)  [unwired: 1 in]
        n129 = case shown="\"Tune Buck-Boost\"" w318 {
          tunnel: w322 -> [_ w348 w364 w392]
          tunnel: [w323 w329 w354 w381] -> w321
          tunnel: w320 -> [_ w347 w363 w391]
          tunnel: w319 -> [w323 w346 w362 w390]
          frame Default {
          }
          frame "Tune PLL" {
            w326 = T3 {"output high (Inf)"=inf, "output low (-Inf)"=-inf} ("data")
            w335 = T4 {"proportional gain"=0.0, "integral gain"=0.0} ("PLL Gains")
            n130 = call "RequestAndTrace.vi"("JSONRef in"=w348, "TraceRef"=w347, "method"="PllSettings" ("resulting string"), "error in (no error)"=w346) -> ("reponse"=w344:string, "error out"=w345:errorcluster)  [unwired: 9 in, 1 out]
            n131 = call <vilib>:"From String.vi"("error in (no error)"=w345, "JSON String"=w344) -> ("error out"=w343:errorcluster, "JSON out"=w341:refnum<class "JSON Null.lvclass">)  [unwired: 8 in]
            n132 = call-poly <vilib>:"To More Specific Type.vi"("error in (no error)"=w343, "JSON Datatype in"=w341) -> ("error out"=w342:errorcluster, "JSON Datatype out"=w340:refnum<class "JSON Object.lvclass">)  [unwired: 8 in]
            n133 = call-poly <vilib>:"Get Parameter Value.vi"("error in (no error)"=w342, "Keys"=string[] ["result", "PI", "PLLgains"], "JSON Object in"=w340) -> ("error out"=w339:errorcluster, "JSON Object out"=w338:refnum<class "JSON Object.lvclass">)  [unwired: 7 in]
            n134 = call <vilib>:"To Variant.vi"("error in (no error)"=w339, "datatype and defaults"=w335, "JSON Datatype in"=w338) -> ("error out"=w337:errorcluster, "Variant"=w336:variant)  [unwired: 6 in, 1 out]
            n135 = Variant To Data(error in=w337, type=w335, Variant=w336) -> (data=w334:T4, error out=w333:errorcluster)
            n136 = local write "PLL Gains"(w334) -> ()
            n137 = call-poly <vilib>:"Get Parameter Value.vi"("error in (no error)"=w333, "Keys"=string[] ["result", "PI", "PLLrange"], "JSON Object in"=w340) -> ("error out"=w330:errorcluster, "JSON Object out"=w331:refnum<class "JSON Object.lvclass">)  [unwired: 7 in]
            n138 = call <vilib>:"To Variant.vi"("error in (no error)"=w330, "datatype and defaults"=w326, "JSON Datatype in"=w331) -> ("error out"=w332:errorcluster, "Variant"=w328:variant)  [unwired: 6 in, 1 out]
            n139 = Variant To Data(error in=w332, type=w326, Variant=w328) -> (data=w327:T3, error out=w329:errorcluster)
            n140 = local write "PLL Range"(w327) -> ()
          }
          frame "Tune AFE" {
            n141 = call "RequestAndTrace.vi"("JSONRef in"=w364, "TraceRef"=w363, "method"="AfeSettings" ("resulting string"), "error in (no error)"=w362) -> ("reponse"=w360:string, "error out"=w361:errorcluster)  [unwired: 9 in, 1 out]
            n142 = call <vilib>:"From String.vi"("error in (no error)"=w361, "JSON String"=w360) -> ("error out"=w359:errorcluster, "JSON out"=w358:refnum<class "JSON Null.lvclass">)  [unwired: 8 in]
            n143 = call-poly <vilib>:"To More Specific Type.vi"("error in (no error)"=w359, "JSON Datatype in"=w358) -> ("error out"=w357:errorcluster, "JSON Datatype out"=w356:refnum<class "JSON Object.lvclass">)  [unwired: 8 in]
            n144 = for {
              shift-right: [w366] -> _
              shift-left: w356 -> [w366]
              shift-right: [w368] -> w354
              shift-left: w357 -> [w375]
              tunnel: string[][] [["result", "IDtoVD"], ["result", "IQtoVQ"], ["result", "VDCLinkToPower"]] -> [w374] mode=indexing
              tunnel: [w367] -> w353 mode=indexing
              w369 = T5 {"gains"={"proportional gain"=0.0, "integral gain"=0.0}, "output range"={"output high (Inf)"=inf, "output low (-Inf)"=-inf}, "PI_state"=enum."idle", "reset"=FALSE, "manual"=0.0} ("ID_to_VD")
              n145 = call-poly <vilib>:"Get Parameter Value.vi"("error in (no error)"=w375, "Keys"=w374, "JSON Object in"=w366) -> ("error out"=w373:errorcluster, "JSON Object out"=w372:refnum<class "JSON Object.lvclass">)  [unwired: 7 in]
              n146 = call <vilib>:"To Variant.vi"("error in (no error)"=w373, "datatype and defaults"=w369, "JSON Datatype in"=w372) -> ("error out"=w371:errorcluster, "Variant"=w370:variant)  [unwired: 6 in, 1 out]
              n147 = Variant To Data(error in=w371, type=w369, Variant=w370) -> (data=w367:T5, error out=w368:errorcluster)
            }
            n148 = Index Array(array=w353) -> (element #1=w352:T5, element #2=w351:T5, element #3=w350:T5)  [unwired: 3 in]
            n149 = local write "ID_to_VD"(w352) -> ()
            n150 = local write "IQ_to_VQ"(w351) -> ()
            n151 = local write "VDCLinkToPower"(w350) -> ()
          }
          frame "Tune Buck-Boost" {
            w383 = T6 {"gains"={"proportional gain"=0.0, "integral gain"=0.0}, "manualInput"=0.0, "rampRate"=0.0, "pertAmp"=0.0, "pertFreq"=0.0, "controlFreq"=0.0, "state"=enum."disabled"} ("Buck-Boost Tune")
            n152 = call "RequestAndTrace.vi"("JSONRef in"=w392, "TraceRef"=w391, "method"="BuckBoostSettings" ("resulting string"), "error in (no error)"=w390) -> ("reponse"=w388:string, "error out"=w389:errorcluster)  [unwired: 9 in, 1 out]
            n153 = call <vilib>:"From String.vi"("error in (no error)"=w389, "JSON String"=w388) -> ("error out"=w387:errorcluster, "JSON out"=w386:refnum<class "JSON Null.lvclass">)  [unwired: 8 in]
            n154 = call-poly <vilib>:"To More Specific Type.vi"("error in (no error)"=w387, "JSON Datatype in"=w386) -> ("error out"=w379:errorcluster, "JSON Datatype out"=w380:refnum<class "JSON Object.lvclass">)  [unwired: 8 in]
            n155 = call-poly <vilib>:"Get Parameter Value.vi"("error in (no error)"=w379, "key"="result", "JSON Object in"=w380) -> ("error out"=w376:errorcluster, "value"=w377:refnum<class "JSON Object.lvclass">)  [unwired: 7 in]
            n156 = call <vilib>:"To Variant.vi"("error in (no error)"=w376, "datatype and defaults"=w383, "JSON Datatype in"=w377) -> ("error out"=w385:errorcluster, "Variant"=w384:variant)  [unwired: 6 in, 1 out]
            n157 = Variant To Data(error in=w385, type=w383, Variant=w384) -> (data=w382:T6, error out=w381:errorcluster)
            n158 = local write "BuckBoostTune"(w382) -> ()
          }
        }
      }
      event "Exit": Value Change {
        n159 = event-data() -> ()  [unwired: 1 in, 1 out]
      }
    }
    n160 = global read "client_globals.vi" "exit"() -> (w50:bool)
    n161 = call "Specific Error Handler"("Error to Check"=w49) -> ("error out"=w48:errorcluster)  [unwired: 11 in, 3 out]
    n162 = Select(t=w43, s=w41, f=w42) -> (s? t:f=w44:T12)
  }
  n163 = case shown="No Error" w21 {
    frame No Error {
      n164 = while {
        stop <- w399 stop-if-true
        n165 = call <userlib>:"SEH Get Next Error.vi"() -> ("Transmission Error"=w395:errorcluster, "Transmitted Error"=w398:errorcluster, "Empty?"=w397:bool, "Notification Info"=w396:T15)  [unwired: 8 in]
        n166 = case shown="False" w397 {
          tunnel: [w408 w425] -> w400
          tunnel: w398 -> [w407 _]
          tunnel: w396 -> [w403 _]
          tunnel: [w402 FALSE] -> w399
          tunnel: w395 -> [_ _]
          frame False {
            w408 = u32 1  # Prevents a continuous stream of errors from starving the processor
            n167 = call <userlib>:"De-Classify Error.vi"("Classified Error"=w407) -> ("De-Classified Error"=w405:errorcluster, "Error Classification"=w406:string)  [unwired: 8 in, 1 out]
            n168 = case shown="\"Critical Error\"" w406 {
              tunnel: [w409 w410 w411 w412 w413 w414] -> w404
              frame "Exit" {
                w409 = T16[] [enum."Log", enum."Shutdown"] items=["Log", "Display Error Message", "Safe State", "Shutdown"]
              }
              frame Default {
                w410 = T16[] [enum."Log", enum."Display Error Message", enum."Safe State", enum."Shutdown"] items=["Log", "Display Error Message", "Safe State", "Shutdown"]
                # "Un-classified erorr or\nUn-recognized classification"
              }
              frame "Warning" {
                w411 = T16[] [enum."Log"] items=["Log", "Display Error Message", "Safe State", "Shutdown"]
              }
              frame "Invalid Input" {
                w412 = T16[] [enum."Display Error Message"] items=["Log", "Display Error Message", "Safe State", "Shutdown"]
              }
              frame "IO Error" {
                w413 = T16[] [enum."Log", enum."Safe State"] items=["Log", "Display Error Message", "Safe State", "Shutdown"]
              }
              frame "Critical Error" {
                w414 = T16[] [enum."Log", enum."Safe State", enum."Shutdown"] items=["Log", "Display Error Message", "Safe State", "Shutdown"]
              }
            }
            n169 = for {
              tunnel: w405 -> [w419]
              tunnel: w404 -> [w420] mode=indexing
              tunnel: w403 -> [w418]
              border: FALSE -> [_]
              tunnel: [w415] -> w402
              n170 = case shown="\"Shutdown\"" w420 {
                tunnel: w419 -> [_ w421 _ _]
                tunnel: w418 -> [_ _ _ _]
                tunnel: [_ _ _ TRUE] -> w417
                frame "Log", Default {
                  # "Implement log \nhere"
                }
                frame "Display Error Message" {
                  n171 = call <vilib>:"Simple Error Handler.vi"("error in (no error)"=w421) -> ()  [unwired: 4 in, 5 out]
                }
                frame "Safe State" {
                  # "Implement safe\nstate here"
                }
                frame "Shutdown" {
                  n172 = global write "client_globals.vi" "exit"(TRUE ("exit")) -> ()
                }
              }
              n173 = feedback #1() -> (w416:bool)
              n174 = Or(x=w417, y=w416) -> (x .or. y?=w415:bool)
              n175 = feedback-in #1(w415) -> ()
            }
          }
          frame True {
            w425 = u32 10  # Error poll period
          }
        }
        n176 = Wait (ms)(milliseconds to wait=w400) -> ()  [unwired: 1 out]
      }
    }
    frame Error {
      # "Error notification cannot initialize\n(log this)"
    }
  }
  n177 = while {
    shift-right: [w439] -> _
    shift-left: StreamClientState."Initialize" ("StreamClientState") -> [w440]
    shift-right: [w437] -> w17
    shift-left: _ -> [w436]
    shift-right: [w435] -> _
    shift-left: T9 {"Channels"=[], "SampleRate"=0} ("StreamHeader") -> [w434]
    tunnel: w25 -> [w432]
    shift-right: [w426] -> _
    shift-left: _ -> [w431]
    shift-right: [w428] -> w16
    shift-left: _ -> [w427]
    tunnel: w20 -> [w438]
    tunnel: [w429] -> _
    stop <- w433 stop-if-true
    n178 = case shown="\"ConnectAndOpen\"" w440 {
      tunnel: [StreamClientState."Idle" ("StreamClientState") w464 w508 w544 w565 w609 StreamClientState."Idle" ("StreamClientState")] -> w439
      tunnel: w438 -> [w443 w460 w504 w543 w577 w630 _]
      tunnel: [w451 w455 w495 w535 w566 w610 w639] -> w430
      tunnel: [refnum<k5> refnum ("connection ID") refnum<k5> refnum ("connection ID") w506 w545 w568 w620 refnum<k5> refnum ("connection ID")] -> w437
      tunnel: w436 -> [_ _ _ _ w576 w629 w652]
      tunnel: [T9 {"Channels"=[], "SampleRate"=0} ("StreamHeader") T9 {"Channels"=[], "SampleRate"=0} ("StreamHeader") _ _ w553 w616 _] -> w435
      tunnel: w434 -> [_ _ _ _ _ w616 _]
      tunnel: w432 -> [_ w461 _ _ _ w608 _]
      tunnel: [FALSE w454 w507 w542 w557 w613 FALSE] -> w426
      tunnel: w431 -> [_ _ w507 w542 w557 w613 _]
      tunnel: [refnum<k34> refnum ("tdms file out") refnum<k34> refnum ("tdms file out") w500 refnum<k34> refnum ("tdms file out") w555 w612 refnum<k34> refnum ("tdms file out")] -> w428
      tunnel: w427 -> [_ _ _ _ w556 w612 w646]
      frame "Initialize" {
        n179 = property on="StreamAndLog" class="Bool"(error in=w443, "DisabledEnum"=T11."Enabled" ("Disabled")) -> (error out=w445:errorcluster)  [unwired: 1 in, 1 out]
        n180 = property on="Stream" class="Bool"(error in=w445, "DisabledEnum"=T11."Enabled" ("Disabled")) -> (error out=w447:errorcluster)  [unwired: 1 in, 1 out]
        n181 = property on="StopStreaming" class="Bool"(error in=w447, "DisabledEnum"=T11."Disabled and Grayed Out" ("Disabled")) -> (error out=w451:errorcluster)  [unwired: 1 in, 1 out]
      }
      frame "Idle", Default {
        n182 = Dequeue Element(queue=w461, timeout in ms (-1)=100, error in (no error)=w460) -> (element=w457:T8, timed out?=w458:bool, error out=w456:errorcluster)  [unwired: 1 out]
        n183 = case shown="False" w458 {
          tunnel: [w473 StreamClientState."Idle" ("StreamClientState")] -> w464
          tunnel: w457 -> [w472 _]
          tunnel: w456 -> [w470 w489]
          tunnel: [w467 w489] -> w455
          tunnel: [w465 FALSE] -> w454
          frame False {
            n184 = Unbundle By Name(w472) -> ("cmd"=w471:string)
            n185 = case shown="\"StartStream\"" w471 {
              selector: w471 -> [w478 _ _]
              tunnel: [StreamClientState."Idle" ("StreamClientState") StreamClientState."Connecting" ("StreamClientState") StreamClientState."ConnectAndOpen" ("StreamClientState")] -> w473
              tunnel: w470 -> [w475 w481 w486]
              tunnel: [w476 "Starting to stream" "Starting to log streaming data"] -> w468
              tunnel: [w475 w481 w486] -> w466
              tunnel: [FALSE FALSE TRUE] -> w465
              frame Default {
                n186 = Concatenate Strings(w478, " command ignored" ("string")) -> (w476:string)
              }
              frame "StartStream" {
              }
              frame "StartStreamAndLog" {
              }
            }
            n187 = control-ref of="Trace"() -> (w469:refnum<vi>)
            n188 = call "ToTrace.vi"("ToTrace"=w468, "TraceRef"=w469, "error in (no error)"=w466) -> ("error out"=w467:errorcluster)  [unwired: 12 in]
          }
          frame True {
          }
        }
      }
      frame "ConnectAndOpen" {
        w494 = T11."Disabled and Grayed Out" ("Disabled")
        w499 = "*.tdms" ("pattern label")
        n189 = local read "Connection"() -> (w492:T1)
        n190 = Unbundle By Name(w492) -> ("ip"=w491:string)
        n191 = call "File Dialog"("prompt"="Select a new stream fie location", "error in"=w504, "pattern (all files)"=w499, "pattern label"=w499) -> ("selected path"=w501:path, "cancelled"=w502:bool, "error out"=w503:errorcluster)  [unwired: 8 in, 1 out]
        n192 = case shown="False" w502 {
          tunnel: [w521 errorcluster {"status"=FALSE, "code"=0, "source"=""} ("error IO")] -> w498
          tunnel: [w520 StreamClientState."Disconnecting" ("StreamClientState")] -> w508
          tunnel: w491 -> [w519 _]
          tunnel: [w518 refnum<k5> refnum ("connection ID")] -> w506
          tunnel: w503 -> [w517 _]
          tunnel: w501 -> [w515 _]
          tunnel: [w512 _] -> w500
          frame False {
            n193 = TDMS Open(5:FALSE ("create index file? (T)"), 8:w517, 10:T17."create or replace" ("operation (0:open)"), 11:w515) -> (0:w516:errorcluster, 3:w512:refnum<k34>)  [unwired: 3 in]
            n194 = TCP Open Connection(address=w519, remote port or service name=u16 55550, timeout ms (60000)=5000, error in (no error)=w516) -> (connection ID=w518:refnum<k5>, error out=w510:errorcluster)  [unwired: 1 in]
            n195 = Unbundle By Name(w510) -> ("code"=w509:i32)
            n196 = case shown="0" w509 {
              tunnel: [w524 w526] -> w521
              tunnel: [StreamClientState."ReadHeader" ("StreamClientState") StreamClientState."Disconnecting" ("StreamClientState")] -> w520
              tunnel: w510 -> [w524 w526]
              frame 0 {
                n197 = One Button Dialog(message="Unable to connect. Check connection settings.") -> ()  [unwired: 1 in, 1 out]
              }
              frame Default {
              }
            }
          }
          frame True {
          }
        }
        n198 = property on="Stream" class="Bool"(error in=w498, "DisabledEnum"=w494) -> (error out=w497:errorcluster)  [unwired: 1 in, 1 out]
        n199 = property on="StreamAndLog" class="Bool"(error in=w497, "DisabledEnum"=w494) -> (error out=w496:errorcluster)  [unwired: 1 in, 1 out]
        n200 = property on="StopStreaming" class="Bool"(error in=w496, "DisabledEnum"=T11."Enabled" ("Disabled")) -> (error out=w495:errorcluster)  [unwired: 1 in, 1 out]
      }
      frame "Connecting" {
        w538 = T11."Disabled and Grayed Out" ("Disabled")
        n201 = local read "Connection"() -> (w534:T1)
        n202 = Unbundle By Name(w534) -> ("ip"=w533:string)
        n203 = TCP Open Connection(address=w533, remote port or service name=u16 55550, timeout ms (60000)=5000, error in (no error)=w543) -> (connection ID=w545:refnum<k5>, error out=w531:errorcluster)  [unwired: 1 in]
        n204 = Unbundle By Name(w531) -> ("code"=w532:i32)
        n205 = case shown="63, Default" w532 {
          tunnel: [w548 w551] -> w539
          tunnel: [StreamClientState."ReadHeader" ("StreamClientState") StreamClientState."Disconnecting" ("StreamClientState")] -> w544
          tunnel: w531 -> [w548 w551]
          frame 0 {
          }
          frame 63, Default {
            n206 = One Button Dialog(message="Unable to connect. Check connection settings.") -> ()  [unwired: 1 in, 1 out]
          }
        }
        n207 = property on="Stream" class="Bool"(error in=w539, "DisabledEnum"=w538) -> (error out=w540:errorcluster)  [unwired: 1 in, 1 out]
        n208 = property on="StreamAndLog" class="Bool"(error in=w540, "DisabledEnum"=w538) -> (error out=w537:errorcluster)  [unwired: 1 in, 1 out]
        n209 = property on="StopStreaming" class="Bool"(error in=w537, "DisabledEnum"=T11."Enabled" ("Disabled")) -> (error out=w535:errorcluster)  [unwired: 1 in, 1 out]
      }
      frame "ReadHeader" {
        w569 = 1000 ("timeout ms (25000)")
        n210 = TCP Read(connection ID=w576, bytes to read=4, error in (no error)=w577, 9:w569) -> (connection ID out=w571:refnum<k5>, data out=w574:string, error out=w572:errorcluster)  [unwired: 1 in]
        n211 = Type Cast(type=0, x=w574) -> (*(type *) &x=w570:i32)
        n212 = TCP Read(connection ID=w571, bytes to read=w570, error in (no error)=w572, 9:w569) -> (connection ID out=w568:refnum<k5>, data out=w564:string, error out=w567:errorcluster)  [unwired: 1 in]
        n213 = Unflatten From String(type=T9 {"Channels"=[], "SampleRate"=0} ("StreamHeader"), binary string=w564) -> (value=w553:T9)  [unwired: 3 in, 2 out]
        n214 = Unbundle By Name(w553) -> ("SampleRate"=w554:i32)
        n215 = Get Date/Time In Seconds() -> (seconds since 1Jan1904=w561:timestamp)
        n216 = Reciprocal(x=w554) -> (1/x=w562:dbl)
        n217 = To Variant(anything=w561) -> (Variant=w559:variant)
        n218 = To Variant(anything=w562) -> (Variant=w560:variant)
        n219 = Build Array(w560, w559) -> (w558:variant[])
        n220 = case shown="No Error" w567 {
          selector: w567 -> [w579 w601]
          tunnel: [w586 w601] -> w566
          tunnel: [StreamClientState."Streaming" ("StreamClientState") StreamClientState."Disconnecting" ("StreamClientState")] -> w565
          tunnel: w556 -> [w585 w600]
          tunnel: [w584 w600] -> w555
          tunnel: w558 -> [w583 _]
          tunnel: w557 -> [w582 _]
          tunnel: w553 -> [w581 _]
          frame No Error {
            n221 = Unbundle By Name(w581) -> ("Channels"=w580:string[])
            n222 = for {
              tunnel: w580 -> [w590] mode=indexing
              shift-right: [w588] -> w578
              shift-left: w579 -> [w589]
              i -> [w591]
              n223 = property on="Waveforms" class="WFGraph (strict)"(error in=w589, "Active Plot"=w591, "Plot.Plot Name"=w590) -> (error out=w588:errorcluster)  [unwired: 1 in, 1 out]
            }
            n224 = case shown="True" w582 {
              tunnel: w578 -> [w592 w599]
              tunnel: [w592 w598] -> w586
              tunnel: w585 -> [w593 w597]
              tunnel: [w593 w596] -> w584
              tunnel: w583 -> [_ w594]
              frame False {
              }
              frame True {
                n225 = TDMS Set Properties(5:w594, 7:string[] ["wf_increment", "wf_start_time"] ("property names"), 8:w599, 11:w597) -> (0:w598:errorcluster, 3:w596:refnum<k34>)  [unwired: 2 in, 2 out]
              }
            }
          }
          frame Error {
          }
        }
      }
      frame "Streaming" {
        w622 = 1000 ("timeout ms (25000)")
        n226 = Dequeue Element(queue=w608, timeout in ms (-1)=0) -> (element=w605:T8, error out=w606:errorcluster)  [unwired: 1 in, 2 out]
        n227 = Unbundle By Name(w605) -> ("cmd"=w604:string)
        n228 = case shown="\"\"" w604 {
          tunnel: w606 -> [_ _ _]
          tunnel: [StreamClientState."Streaming" ("StreamClientState") StreamClientState."Streaming" ("StreamClientState") StreamClientState."Disconnecting" ("StreamClientState")] -> w603
          frame Default {
          }
          frame "" {
          }
          frame "StopStream" {
          }
        }
        n229 = TCP Read(connection ID=w629, bytes to read=4, error in (no error)=w630, 9:w622) -> (connection ID out=w624:refnum<k5>, data out=w627:string, error out=w625:errorcluster)  [unwired: 1 in]
        n230 = Type Cast(type=0, x=w627) -> (*(type *) &x=w623:i32)
        n231 = TCP Read(connection ID=w624, bytes to read=w623, error in (no error)=w625, 9:w622) -> (connection ID out=w620:refnum<k5>, data out=w621:string, error out=w617:errorcluster)  [unwired: 1 in]
        n232 = Type Cast(type=sgl[] [], x=w621) -> (*(type *) &x=w618:sgl[])
        n233 = call "FormatWaveforms.vi"("WaveformArray"=w618, "logFileRef"=w612, "log"=w613, "StreamHeader"=w616, "error in (no error)"=w617) -> ("Waveforms"=w614:sgl[][], "UpdateWaveforms"=w615:bool, "error out"=w611:errorcluster)  [unwired: 8 in]
        n234 = case shown="True" w615 {
          tunnel: w614 -> [_ w638]
          frame False {
          }
          frame True {
            "Waveforms" <- w638
          }
        }
        n235 = case shown="Error" w611 {
          selector: w611 -> [w635 w637]
          tunnel: [w635 w637] -> w610
          tunnel: [w634 StreamClientState."Disconnecting" ("StreamClientState")] -> w609
          tunnel: w603 -> [w634 _]
          frame No Error {
          }
          frame Error {
          }
        }
      }
      frame "Disconnecting" {
        w641 = T11."Enabled" ("Disabled")
        n236 = TDMS Close(11:w646) -> (0:w648:errorcluster)  [unwired: 1 in, 1 out]
        n237 = TCP Close Connection(connection ID=w652) -> (error out=w649:errorcluster)  [unwired: 2 in, 1 out]
        n238 = flat-sequence {
          tunnel: w649 -> [_]
          tunnel: w648 -> [_]
          frame #0 {
          }
        }
        n239 = property on="Stream" class="Bool"(error in=errorcluster {"status"=FALSE, "code"=0, "source"=""} ("error IO"), "DisabledEnum"=w641) -> (error out=w644:errorcluster)  [unwired: 1 in, 1 out]
        n240 = property on="StreamAndLog" class="Bool"(error in=w644, "DisabledEnum"=w641) -> (error out=w643:errorcluster)  [unwired: 1 in, 1 out]
        n241 = property on="StopStreaming" class="Bool"(error in=w643, "DisabledEnum"=T11."Disabled and Grayed Out" ("Disabled")) -> (error out=w639:errorcluster)  [unwired: 1 in, 1 out]
      }
    }
    "logging" <- w426
    n242 = global read "client_globals.vi" "exit"() -> (w433:bool)
    n243 = call "Specific Error Handler2"("Error to Check"=w430) -> ("error out"=w429:errorcluster)  [unwired: 11 in, 3 out]
  }
  n244 = flat-sequence {
    tunnel: w1 -> [w654]
    tunnel: w30 -> [_]
    tunnel: w25 -> [w653]
    frame #0 {
      n245 = Release Queue(queue=w653) -> ()  [unwired: 2 in, 3 out]
      n246 = call "Close.vi"("reference in"=w654) -> ()  [unwired: 14 in, 1 out]
    }
  }
  n247 = TDMS Close(11:w16) -> (0:w18:errorcluster)  [unwired: 1 in, 1 out]
  n248 = TCP Close Connection(connection ID=w17) -> (error out=w19:errorcluster)  [unwired: 2 in, 1 out]
  n249 = flat-sequence {
    tunnel: w19 -> [_]
    tunnel: w18 -> [_]
    frame #0 {
    }
  }
